vi "VerifyArguments.vi"(8 "error in (no error)":errorcluster, 11 "ExecuteBuildSpec in":refnum<class "ExecuteBuildSpec.lvclass">) -> (0 "error out":errorcluster, 3 "ExecuteBuildSpec out":refnum<class "ExecuteBuildSpec.lvclass">)   [LabVIEW 2014, in "ExecuteBuildSpec.lvclass"]
uses:
  ExecuteBuildSpec.lvclass
  ExecuteBuildSpec.lvclass/ExecuteBuildSpec.ctl
  Utilities/OperationErrorType.ctl
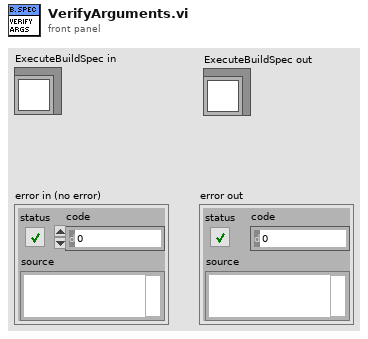
[diagram p1: front panel]
types:
  T1 = typedef "OperationErrorType.ctl" = enum16{"RequiredArgumentMissing", "UnknownArguments", "LoggerSetMultipleTimes", "OperationBrokenError"}
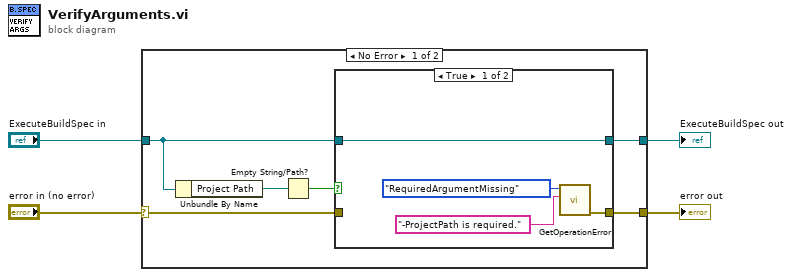
[diagram p0: block diagram]
diagram:
  n1 = case shown="No Error" "error in (no error)" {
    selector: "error in (no error)" -> [w5 w17]
    tunnel: [w10 w17] -> w4
    tunnel: "ExecuteBuildSpec in" -> [w9 w18]
    tunnel: [w8 w18] -> w2
    frame No Error {
      n2 = Unbundle By Name(w9) -> ("Project Path"=w6:path)
      n3 = Empty String/Path?(string/path=w6) -> (empty?=w7:bool)
      n4 = case shown="True" w7 {
        tunnel: w5 -> [_ w16]
        tunnel: [w13 w16] -> w10
        tunnel: w9 -> [w14 w15]
        tunnel: [w14 w15] -> w8
        frame True {
          n5 = call "GetOperationError.vi"("Additional Information"="-ProjectPath is required.", "Operation Error Type"=OperationErrorType."RequiredArgumentMissing") -> ("error out"=w13:errorcluster)  [unwired: 9 in]
        }
        frame False {
        }
      }
    }
    frame Error {
    }
  }
  "error out" <- w4
  "ExecuteBuildSpec out" <- w2
